vi "ColorPatternMatch_MainFunction.vi"(0 "Image in":T4, 5 "Color Pattern Match":T3={"IgnoreBlack And White"=enum."IgnoreBlack And White", "Match Saturation Threshold"=80, "Minimum Match Score"=750, "Color Score Weight"=750, "Color Sensitivity"=1, "Search Strategy"=0, "Match Offset"={"X"=0.0, "Y"=0.0}, "Number of Matches to Find"=1, "AngleRange+/-"=0.0, "Sub-Pixel Accuracy"=FALSE, "ROI Descriptor"={"Global Rectangle"=[], "Contours"=[]}, "TemplatePath"="", "Match Mode"=enum."Shift Invariant"} {"ROI Descriptor"."Contours"."Type" items=["No Selection", "Point", "Line", "Rectangle", "Oval", "Polygon", "Freehand Region", "Annulus", "Unused2", "Unused3", "Broken Line", "Freehand Line", "Rotated Rectangle"]; "Color Score Weight" min=0 max=1000; "Search Strategy" items=["Conservative", "Balance", "Aggressive", "VeryAggressive"]; "Minimum Match Score" min=0 max=1000; "Color Sensitivity" items=["Low", "Medium", "High"]; "Match Saturation Threshold" min=10 max=255 step=1}, 7 "ROI Descriptor":T1 {"Contours"."Type" items=["No Selection", "Point", "Line", "Rectangle", "Oval", "Polygon", "Freehand Region", "Annulus", "Unused2", "Unused3", "Broken Line", "Freehand Line", "Rotated Rectangle"]}, 11 "error in":errorcluster) -> (4 "Image Out":T4(plugin-control), 6 "Matches out":T2(array[cluster]) {"Bounding Box"."y" format="%.2f"; "Bounding Box"."x" format="%.2f"; "Position"."y" format="%.2f"; "Position"."x" format="%.2f"; "Score" format="%.2f"; "Scale" format="%.2f"; "Angle" format="%.2f"}, 8 "Number of Matches":i32, 10 "Calibrated Matches":T2(array[cluster]) {"Bounding Box"."y" format="%.2f"; "Bounding Box"."x" format="%.2f"; "Position"."y" format="%.2f"; "Position"."x" format="%.2f"; "Score" format="%.2f"; "Scale" format="%.2f"; "Angle" format="%.2f"}, 15 "error out":errorcluster)   [LabVIEW 2019]
uses:
  <vilib>/vision/Image Controls.llb/IMAQ Image.ctl
  Controls/Color Pattern Match/Analysis Color Pattern Match Parameter.ctl
  <vilib>/vision/NI_Vision_Development_Module.lvlib
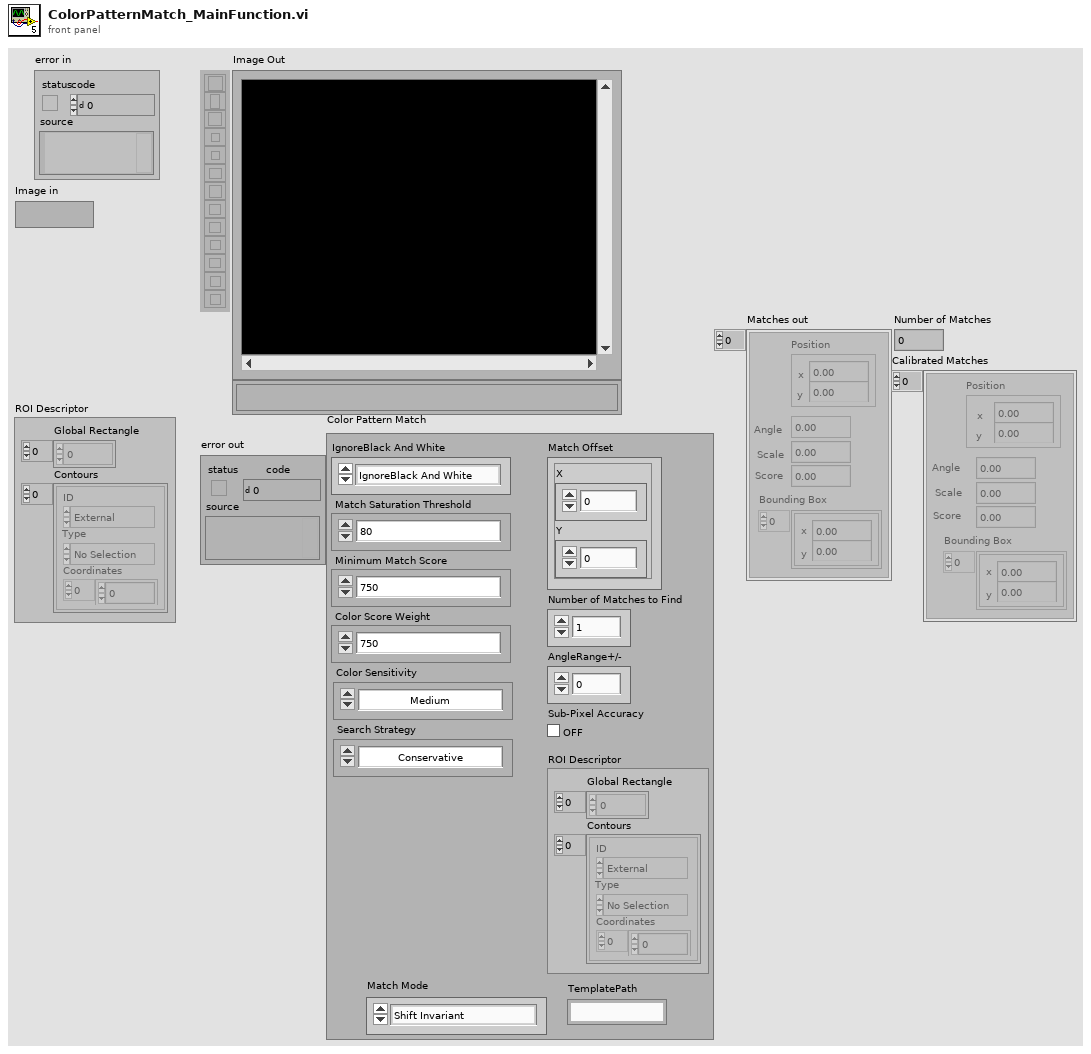
[diagram p1: front panel]
types:
  T1 = typedef "ROI Descriptor" = cluster{"Global Rectangle":i32[], "Contours":cluster{"ID":enum32{"External", "Internal"}, "Type":u32, "Coordinates":i32[]}[]}
  T2 = cluster{"Position":cluster{"x":sgl, "y":sgl}, "Angle":sgl, "Scale":sgl, "Score":sgl, "Bounding Box":cluster{"x":sgl, "y":sgl}[]}[]
  T3 = typedef "Analysis Color Pattern Match Parameter.ctl" = cluster{"IgnoreBlack And White":enum16{"Disable", "IgnoreBlack", "IgnoreWhite", "IgnoreBlack And White"}, "Match Saturation Threshold":i32, "Minimum Match Score":i32, "Color Score Weight":i32, "Color Sensitivity":u32, "Search Strategy":u32, "Match Offset":cluster{"X":dbl, "Y":dbl}, "Number of Matches to Find":i32, "AngleRange+/-":dbl, "Sub-Pixel Accuracy":bool, "ROI Descriptor":T1, "TemplatePath":string, "Match Mode":enum16{"Shift Invariant", "Rotation Invariant"}}
  T4 = typedef "IMAQ Image.ctl" = refnum<image>
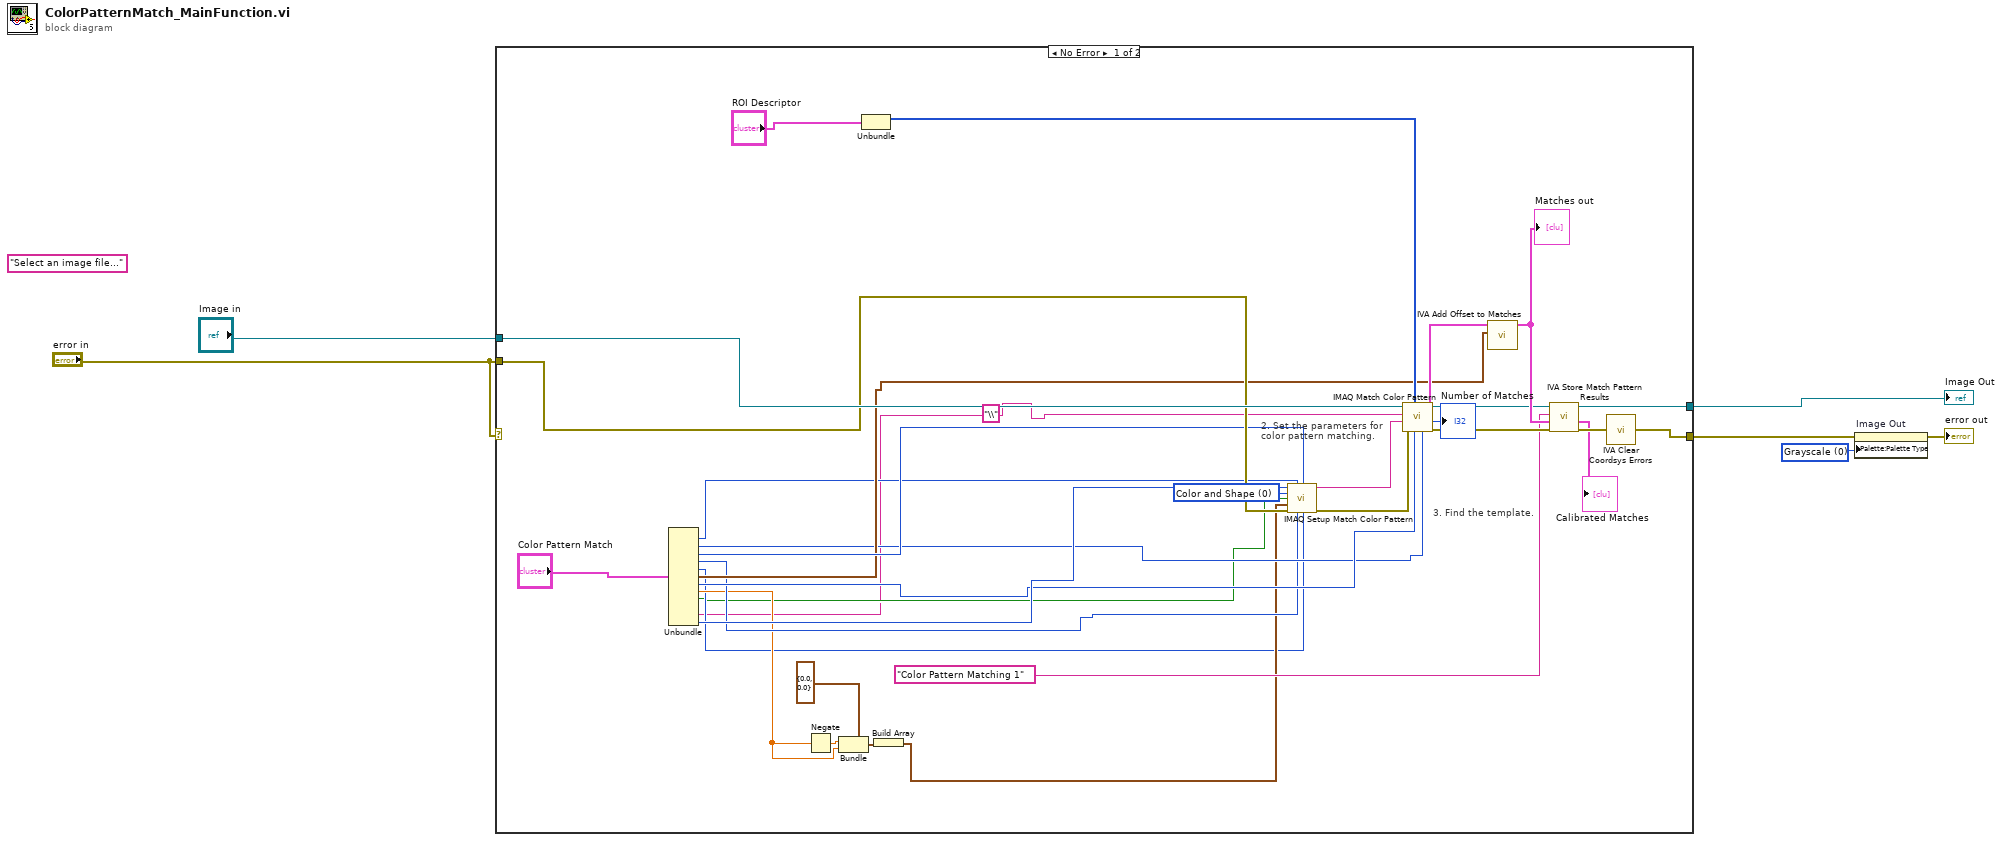
[diagram p0: block diagram]
diagram:
  w3 = u32 0 items=["Grayscale", "Binary", "Gradient", "Rainbow", "Temperature", "User Defined", "Binary 16 Bit", "Gradient 16 Bit", "Rainbow 16 Bit", "Temperature 16 Bit", "User Defined 16 Bit"] ("Palette Type")
  (unwired) "Select an image file..." ("prompt")
  n1 = case shown="No Error" "error in" {
    tunnel: [w30 w39] -> w6
    tunnel: [w29 w40] -> w4
    tunnel: "Image in" -> [w28 w40]
    tunnel: "error in" -> [w27 w39]
    frame No Error {
      (unwired) "\\" ("regular expression")
      w11 = u32 0 items=["Color and Shape", "Color", "Shape"] ("Match Feature Mode")
      # "2. Set the parameters for\ncolor pattern matching."
      # "3. Find the template."
      n2 = Unbundle("Color Pattern Match") -> ("Match Saturation Threshold"=w12:i32, "Minimum Match Score"=w21:i32, "Color Score Weight"=w25:i32, "Color Sensitivity"=w20:u32, "Search Strategy"=w14:u32, "Match Offset"=w23:cluster{"X":dbl, "Y":dbl}, "Number of Matches to Find"=w22:i32, "AngleRange+/-"=w15:dbl, "Sub-Pixel Accuracy"=w13:bool, "TemplatePath"=w9:string, "Match Mode"=w24:enum16{"Shift Invariant", "Rotation Invariant"})  [unwired: 2 out]
      n3 = Negate(x=w15) -> (-x=w16:dbl)
      n4 = Bundle(cluster=cluster{"Min":sgl, "Max":sgl} {"Min"=0.0, "Max"=0.0} ("Angle"), "Min"=w16, "Max"=w15) -> (w18:cluster{"Min":sgl, "Max":sgl})
      n5 = Unbundle("ROI Descriptor") -> ("Global Rectangle"=w32:i32[])  [unwired: 1 out]
      n6 = Build Array(w18) -> (w17:cluster{"Min":sgl, "Max":sgl}[])
      n7 = call "IMAQ Setup Match Color Pattern"("Match Mode"=w24, "Minimum Contrast"=w12, "Color Score Weight"=w25, "Match Feature Mode"=w11, "Subpixel Accuracy"=w13, "Rotation Angle Ranges (degrees)"=w17, "error in (no error)"=w27, "Color Sensitivity"=w20, "Search Strategy"=w14) -> ("Match Color Pattern Setup Data"=w35:string, "error out"=w34:errorcluster)  [unwired: 5 out]
      n8 = call "IMAQ Match Color Pattern"("Minimum Match Score"=w21, "Number of Matches Requested"=w22, "Optional Rectangle"=w32, "error in (no error)"=w34, "Match Color Pattern Setup Data"=w35, "Template Image"=w9, "Image"=w28) -> ("error out"=w37:errorcluster, "Number of Matches"=→"Number of Matches":i32, "Matches"=w33:T2)  [unwired: 2 out]
      n9 = call <vilib>:"IVA Add Offset to Matches.vi"("Match Offset"=w23, "Matches in"=w33) -> ("Matches out"=w38:T2)  [unwired: 9 out]
      "Matches out" <- w38
      n10 = call <vilib>:"IVA Store Match Pattern Results.vi"("error in (no error)"=w37, "Matches"=w38, "Step Name"="Color Pattern Matching 1", "Image in"=w28) -> ("error out"=w31:errorcluster, "Calibrated Matches"=→"Calibrated Matches":T2, "Image dup"=w29:T4)  [unwired: 5 out]
      n11 = call <vilib>:"IVA Clear Coordsys Errors.vi"("error in (no error)"=w31) -> ("error out"=w30:errorcluster)  [unwired: 10 in]
    }
    frame Error {
    }
  }
  "Image Out" <- w4
  n12 = property on="Image Out" class="ImageControl"(error in=w6, "Palette:Palette Type"=w3) -> (error out=→"error out":errorcluster)  [unwired: 1 in, 1 out]
